vi "NC_var_shape.vi"(2 "NC_dimarray":cluster{"name":string, "size":u64}[](array[cluster]), 3 "NC_var in":T1) -> (1 "NC_var out":T1)   [LabVIEW 2016]
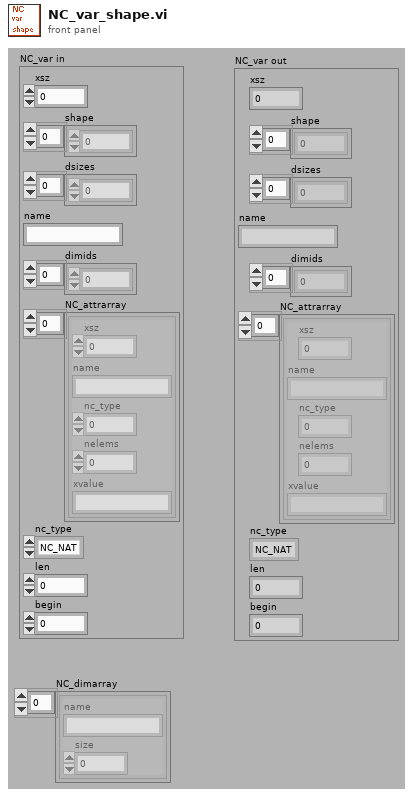
[diagram p1: front panel]
types:
  T1 = cluster{"xsz":u64, "shape":u64[], "dsizes":u64[], "name":string, "dimids":u64[], "NC_attrarray":cluster{"xsz":u64, "name":string, "nc_type":u16, "nelems":u64, "xvalue":string}[], "nc_type":enum16{"NC_NAT", "NC_BYTE", "NC_CHAR", "NC_SHORT", "NC_INT", "NC_FLOAT", "NC_DOUBLE"}, "len":u64, "begin":u64}
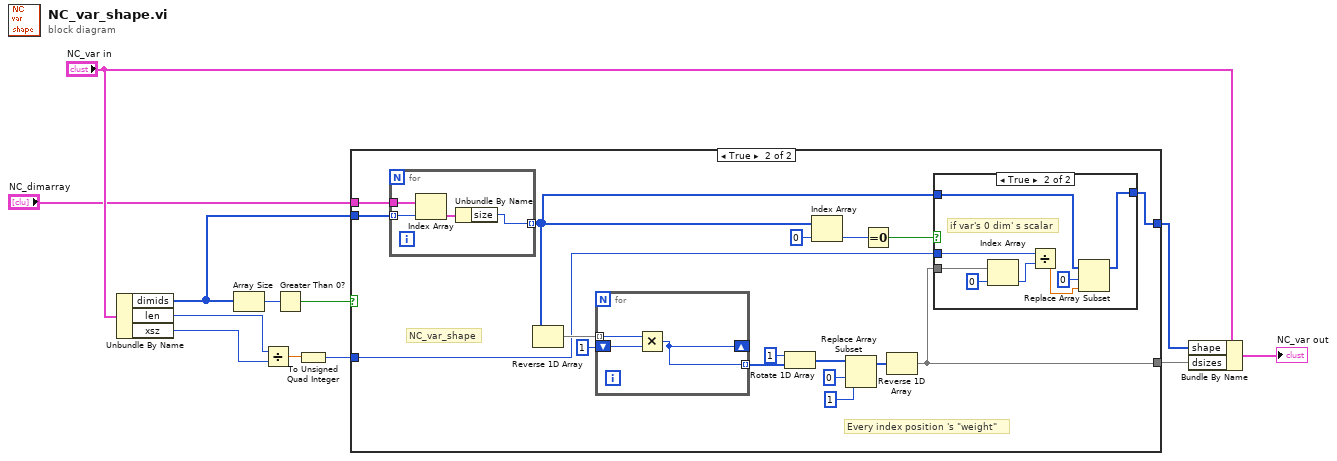
[diagram p0: block diagram]
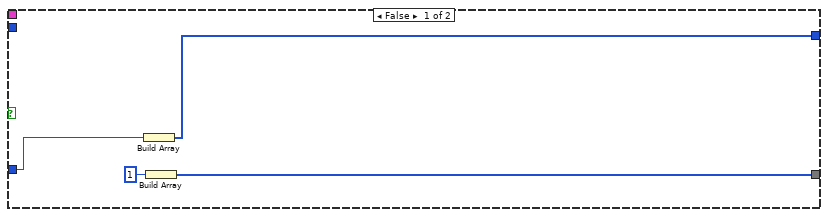
[diagram p2: hidden frame]
diagram:
  n1 = Unbundle By Name("NC_var in") -> ("dimids"=w12:u64[], "len"=w5:u64, "xsz"=w4:u64)
  n2 = Array Size(array=w12) -> (size(s)=w7:i32)
  n3 = Divide(x=w5, y=w4) -> (x/y=w3:dbl)
  n4 = Greater Than 0?(x=w7) -> (x > 0?=w8:bool)
  n5 = To Unsigned Quad Integer(1:w3) -> (0:w2:u64)
  n6 = case shown="True" w8 {
    tunnel: "NC_dimarray" -> [_ w31]
    tunnel: [w16 w17] -> w1
    tunnel: [w14 w20] -> w10
    tunnel: w12 -> [_ w24]
    tunnel: w2 -> [w13 w19]
    frame False {
      n7 = Build Array(w13) -> (w16:u64[])
      n8 = Build Array(u64 1 ("元素")) -> (w14:u64[])
    }
    frame True {
      # "NC_var_shape"
      # "Every index position 's \"weight\""
      n9 = for {
        tunnel: w24 -> [w48] mode=indexing
        tunnel: w31 -> [w49]
        tunnel: [w46] -> w18 mode=indexing
        n10 = Index Array(array=w49, index=w48) -> (element=w47:cluster{"name":string, "size":u64})
        n11 = Unbundle By Name(w47) -> ("size"=w46:u64)
      }
      n12 = Reverse 1D Array(array=w18) -> (reversed array=w32:u64[])
      n13 = for {
        tunnel: w32 -> [w43] mode=indexing
        shift-right: [w44] -> _
        shift-left: u64 1 -> [w45]
        tunnel: [w44] -> w26 mode=indexing
        n14 = Multiply(x=w43, y=w45) -> (x*y=w44:u64)
      }
      n15 = Rotate 1D Array(1:w26, 2:1 ("n")) -> (0:w29:u64[])
      n16 = Index Array(array=w18, index=0 ("索引")) -> (element=w22:u64)
      n17 = Replace Array Subset(array=w29, new element=u64 1 ("索引"), index=0 ("索引")) -> (w25:u64[])
      n18 = Equal To 0?(x=w22) -> (x = 0?=w21:bool)
      n19 = Reverse 1D Array(array=w25) -> (reversed array=w20:u64[])
      n20 = case shown="True" w21 {
        tunnel: w20 -> [_ w41]
        tunnel: w19 -> [_ w40]
        tunnel: w18 -> [w34 w36]
        tunnel: [w34 w35] -> w17
        frame False {
        }
        frame True {
          # "if var's 0 dim' s scalar"
          n21 = Index Array(array=w41, index=0 ("索引")) -> (element=w39:u64)
          n22 = Divide(x=w40, y=w39) -> (x/y=w37:dbl)
          n23 = Replace Array Subset(array=w36, new element=w37, index=0 ("索引")) -> (w35:u64[])
        }
      }
    }
  }
  n24 = Bundle By Name(cluster="NC_var in", "shape"=w1, "dsizes"=w10) -> (→"NC_var out":T1)
